vi "MicroDrive Gamepad.vi"() -> ()   [LabVIEW 2012]
uses:
  <vilib>/Utility/miscctls.llb/LVPointTypeDef.ctl
  <vilib>/Utility/inputDevices.llb/closeJoystick.vi
  <vilib>/Utility/inputDevices.llb/joystickAcquire.vi
  MicroDrive.dll
panel:
  in  "m3f":u16(ring)=6 items=["1 X"=1, "2 A"=2, "3 B"=3, "4 Y"=4, "5 LB"=5, "6 RB"=6, "7 LT"=7, "8 RT"=8, "9 Back"=9]
  in  "m3r":u16(ring)=8 items=["1 X"=1, "2 A"=2, "3 B"=3, "4 Y"=4, "5 LB"=5, "6 RB"=6, "7 LT"=7, "8 RT"=8, "9 Back"=9]
  in  "m1f":u16(ring)=3 items=["1 X"=1, "2 A"=2, "3 B"=3, "4 Y"=4, "5 LB"=5, "6 RB"=6, "7 LT"=7, "8 RT"=8, "9 Back"=9]
  out "button selection refs 2":T1
  out "maxVelocityThreeAxis":dbl
  in  "Invert Z":bool=TRUE
  out "Z rev limt":bool
  out "Z Limit":bool
  in  "m3 f":bool
  in  "m3 b":bool
  in  "M3 Velocity":dbl=1.0 format="%.3f"
  in  "M3 Step":dbl=5.0 step=0.1 format="%_6g"
  in  "Reset M3":bool
  out "M3 Axis":dbl format="%.5f"
  in  "closed?":bool
  in  "Slide":cluster{u32, u32, u32}(slide)={7, 6, 2} scale=0.0..7.0
  in  "configure":bool
  in  "device info":bool
  in  "m2f":u16(ring)=4 items=["1 X"=1, "2 A"=2, "3 B"=3, "4 Y"=4, "5 LB"=5, "6 RB"=6, "7 LT"=7, "8 RT"=8, "9 Back"=9]
  in  "halt 3":u16(ring)=9 items=["1 X"=1, "2 A"=2, "3 B"=3, "4 Y"=4, "5 LB"=5, "6 RB"=6, "7 LT"=7, "8 RT"=8, "9 Back"=9]
  in  "m2r":u16(ring)=2 items=["1 X"=1, "2 A"=2, "3 B"=3, "4 Y"=4, "5 LB"=5, "6 RB"=6, "7 LT"=7, "8 RT"=8, "9 Back"=9]
  in  "m1r":u16(ring)=1 items=["1 X"=1, "2 A"=2, "3 B"=3, "4 Y"=4, "5 LB"=5, "6 RB"=6, "7 LT"=7, "8 RT"=8, "9 Back"=9]
  out "X Limit 2":bool
  out "x rev lim":bool
  out "Y Limit 2":bool
  in  "halt 2":bool
  in  "m1 f 2":bool
  in  "m1 b 2":bool
  in  "m2 f 2":bool
  in  "m2 b 2":bool
  out "Y rev lim":bool
  out "Max Velocity One Axis":dbl
  out "Min Velocity":dbl
  in  "Reset All":bool
  in  "Reset M2":bool
  in  "Reset M1":bool
  in  "M2 Step":dbl=5.0 step=0.1 format="%_6g"
  in  "M1 Step":dbl=5.0 step=0.1 format="%_6g"
  in  "M2 Velocity":dbl=1.0 format="%.3f"
  in  "M1 Velocity":dbl=1.0 format="%.3f"
  out "Max VelocityTwo Axis":dbl format="%.3f"
  in  "Invert":bool=TRUE
  in  "Invert":bool
  out "M2 Axis":dbl format="%.5f"
  out "M1 Axis":dbl format="%.5f"
  # "Single Step Controls"
  # "Current Postion"
  # "Step Distances"
  # "mm"
  # "mm"
  # "mm"
  # "mm"
  # "mm"
  # "mm"
  # "Step Velocities"
  # "mm/s"
  # "mm/s"
  # "mm/s"
  # "M3\nControl"
  # "M1\\M2\nControl"
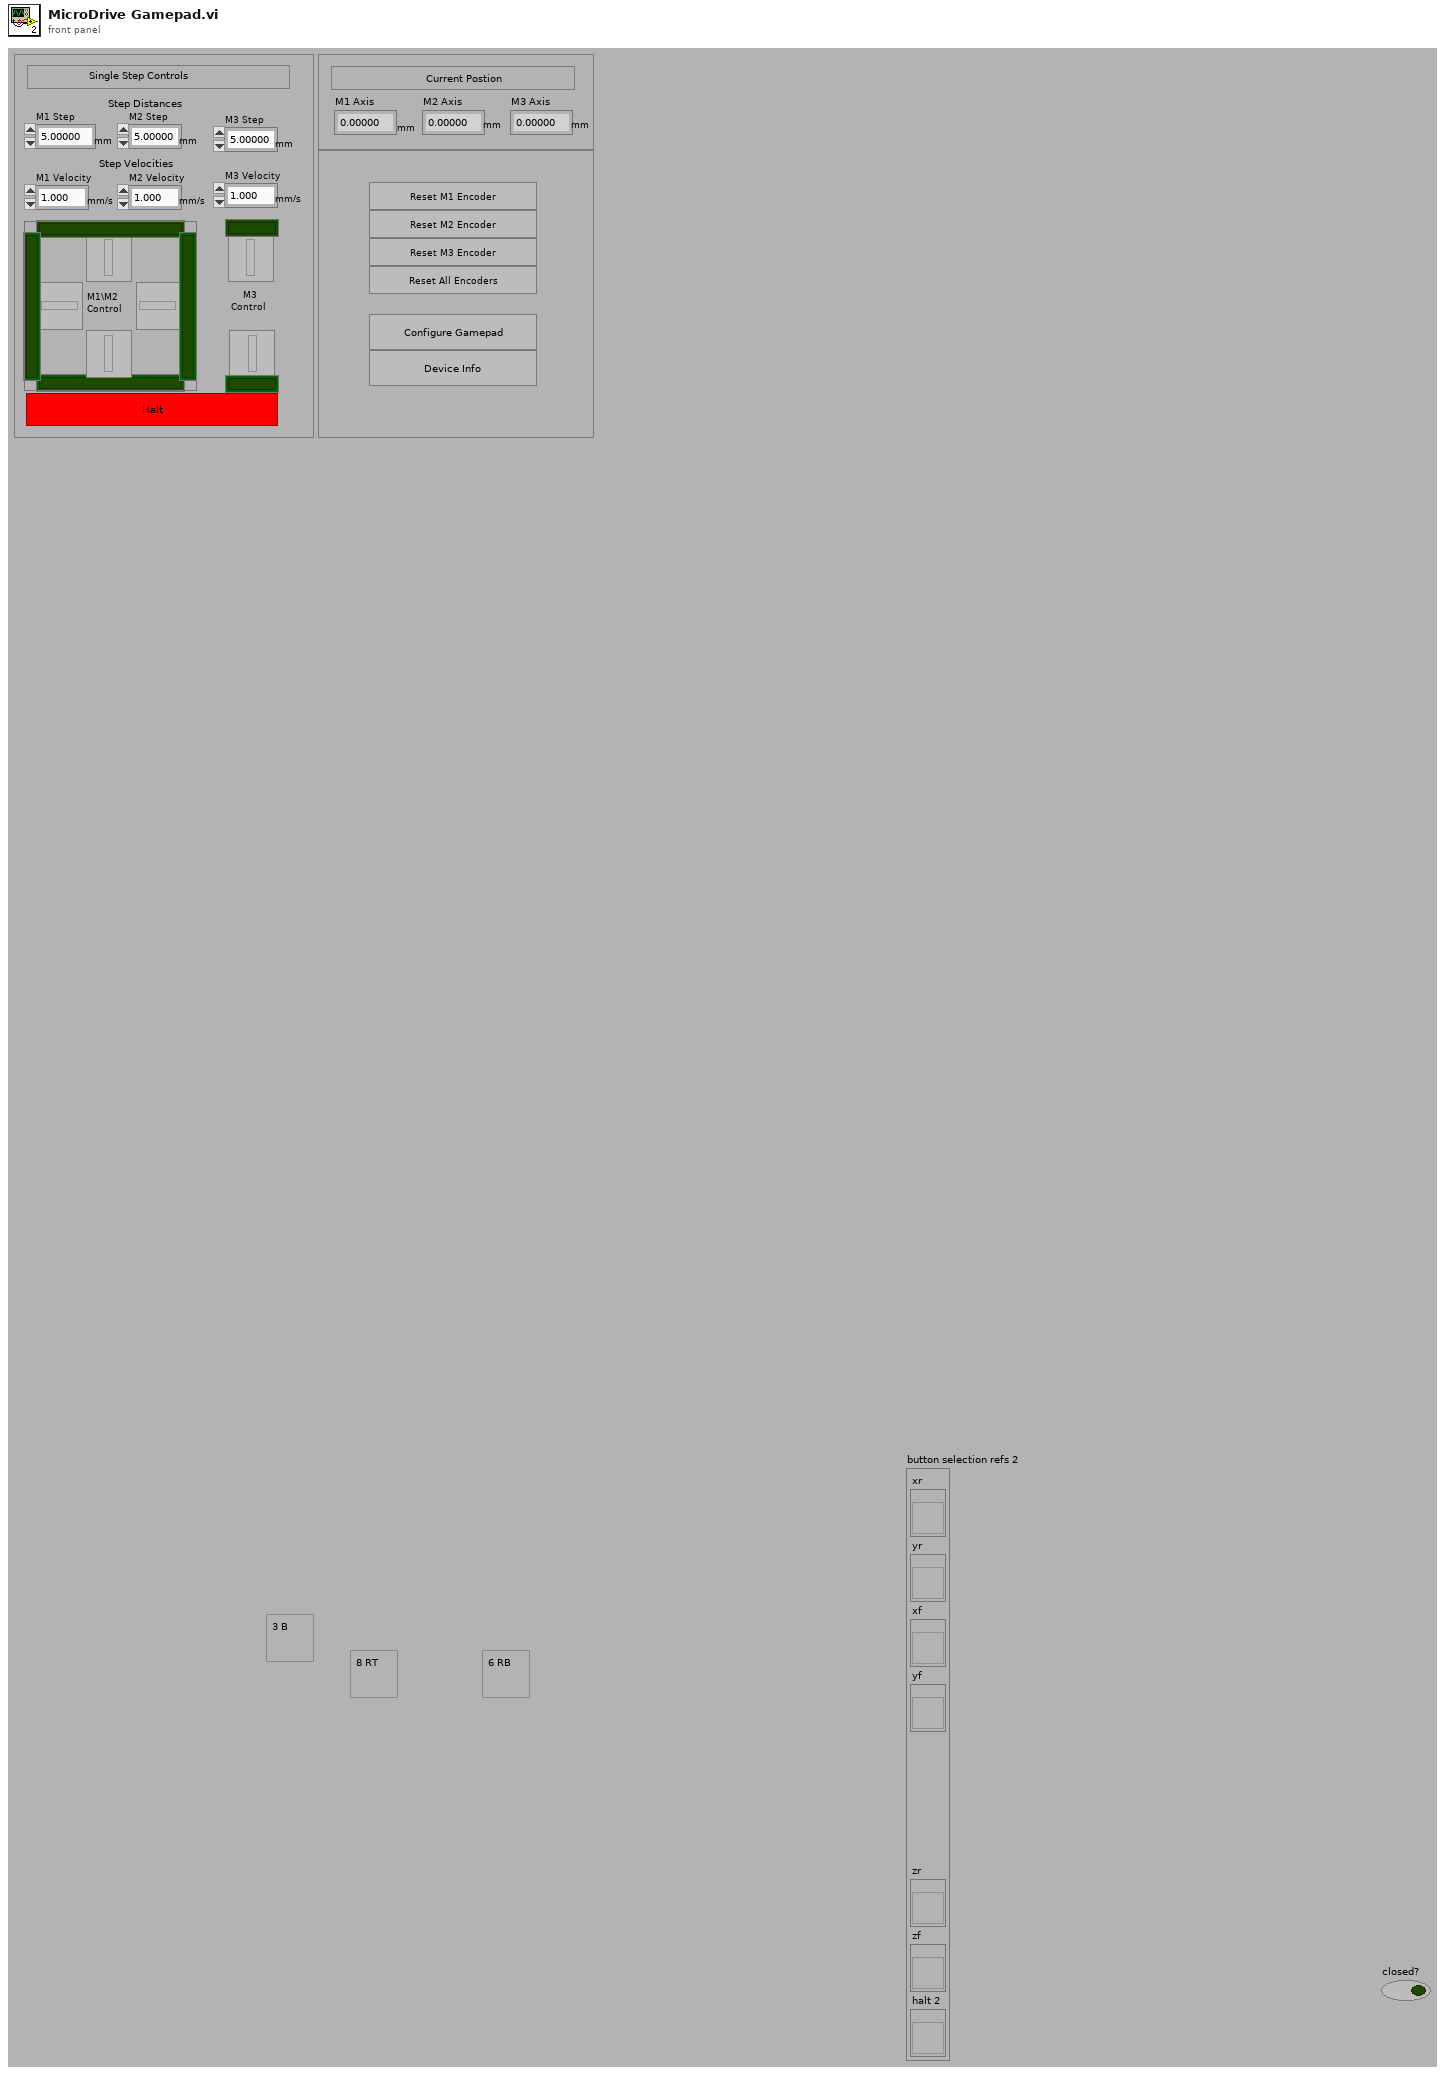
[diagram p1: front panel]
types:
  T1 = cluster{"xr":refnum<vi>, "yr":refnum<vi>, "xf":refnum<vi>, "yf":refnum<vi>, "zr":refnum<vi>, "zf":refnum<vi>, "halt 2":refnum<vi>}
  T2 = typedef "LVPointTypeDef.ctl" = cluster{"Horizontal":i16, "Vertical":i16}
  T3 = cluster{"m1r":refnum<vi>, "m2r":refnum<vi>, "m1f ":refnum<vi>, "m2f":refnum<vi>, "m3r":refnum<vi>, "m3f":refnum<vi>, "halt 3":refnum<vi>}
  T4 = cluster{"X axis":i32, "Y axis":i32, "Z axis":i32, "X axis rotation":i32, "Y axis rotation":i32, "Z axis rotation":i32, "U axis":i32, "V axis":i32}
  T5 = cluster{"button 1":bool, "button 2":bool, "button 3":bool, "button 4":bool, "button 5":bool, "button 6":bool, "button 7":bool, "button 8":bool, "button 9":bool, "button 10":bool, "button 11":bool, "button 12":bool, "button 13":bool, "button 14":bool, "button 15":bool, "button 16":bool, "button 17":bool, "button 18":bool, "button 19":bool, "button 20":bool, "button 21":bool, "button 22":bool, "button 23":bool, "button 24":bool, "button 25":bool, "button 26":bool, "button 27":bool, "button 28":bool, "button 29":bool, "button 30":bool, "button 31":bool, "button 32":bool}
  T6 = cluster{"m1 f 2":bool, "m1 b 2":bool, "m2 f 2":bool, "m2 b 2":bool, "m3 f":bool, "m3 b":bool}
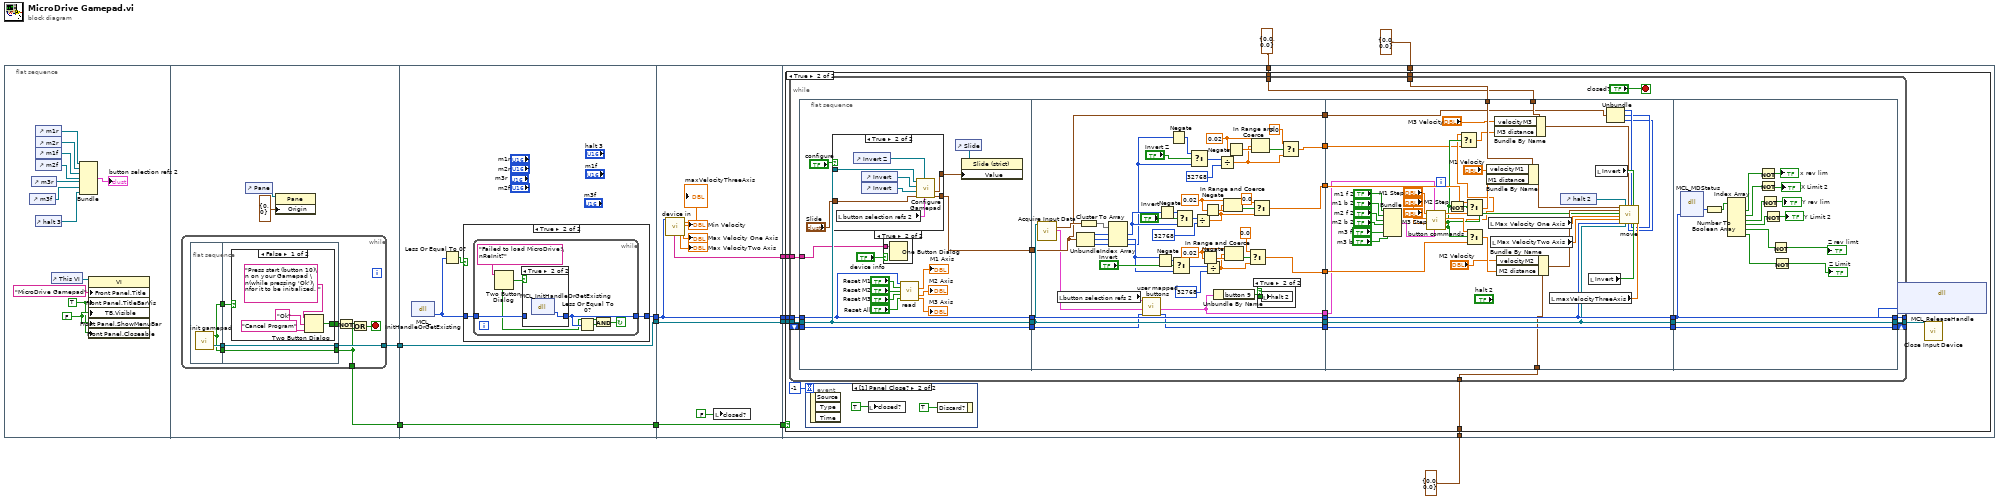
[diagram p0: block diagram]
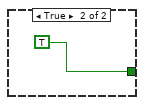
[diagram p2: hidden frame]
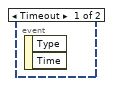
[diagram p6: hidden frame]
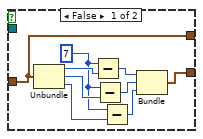
[diagram p8: hidden frame]
diagram:
  n1 = flat-sequence {
    tunnel: [w28] -> w6
    tunnel: [w27] -> w5
    tunnel: [w51] -> w12
    tunnel: [w52] -> w10
    tunnel: [w48] -> w8
    tunnel: w6 -> [w52]
    tunnel: w5 -> [w51]
    tunnel: w12 -> [w71]
    tunnel: [w71] -> w11
    tunnel: w10 -> [w72]
    tunnel: [w72] -> w9
    tunnel: w8 -> [w70]
    tunnel: [w70] -> w7
    tunnel: [w65] -> w4
    tunnel: w7 -> [w77]
    tunnel: w9 -> [w79]
    tunnel: w11 -> [w78]
    tunnel: w4 -> [w76]
    tunnel: cluster{"M1 distance":dbl, "velocityM1":dbl} {"M1 distance"=0.0, "velocityM1"=0.0} ("X Info in") -> [w75]
    tunnel: cluster{"M2 distance":dbl, "velocityM2":dbl} {"M2 distance"=0.0, "velocityM2"=0.0} ("Y Info in") -> [w74]
    tunnel: cluster{"M3 distance":dbl, "velocityM3":dbl} {"M3 distance"=0.0, "velocityM3"=0.0} ("Z Info in") -> [w73]
    frame #0 {
      w18 = TRUE ("Front Panel Window:Closeable")
      w19 = FALSE ("Front Panel Window:Title Bar Visible")
      n2 = control-ref of="m3f"() -> (w13:refnum<vi>)
      n3 = control-ref of="m3r"() -> (w14:refnum<vi>)
      n4 = control-ref of="m1r"() -> (w22:refnum<vi>)
      n5 = control-ref of="m2r"() -> (w23:refnum<vi>)
      n6 = control-ref of="m1f"() -> (w16:refnum<vi>)
      n7 = control-ref of="m2f"() -> (w24:refnum<vi>)
      n8 = control-ref of="halt 3"() -> (w17:refnum<vi>)
      n9 = control-ref of="This VI"() -> (w21:refnum<vi>)
      n10 = Bundle("m1r"=w22, "m2r"=w23, "m1f"=w16, "m2f"=w24, "m3r"=w14, "m3f"=w13, "halt 3"=w17) -> (→"button selection refs 2":T3)  [unwired: 1 out]
      n11 = property class="VI"(reference=w21, "Front Panel.Title"="MicroDrive Gamepad" ("Front Panel Window:Title"), "Front Panel.TitleBarVis"=w18, "TB.Visible"=w19, "Front Panel.ShowMenuBar"=w19, "Front Panel.Closeable"=w18) -> ()  [unwired: 1 in, 2 out]
    }
    frame #1 {
      n12 = while {
        tunnel: [w34] -> w27
        tunnel: [w29] -> w28
        stop <- w33 stop-if-true
        n13 = flat-sequence {
          tunnel: [w37] -> w36
          tunnel: [w38] -> w35
          tunnel: [w37] -> w32
          tunnel: w36 -> [w42]
          tunnel: [w41] -> w34
          tunnel: w35 -> [w41]
          tunnel: [w40] -> w29
          tunnel: w32 -> [w40]
          tunnel: [w39] -> w31
          frame #0 {
            n14 = call "init gamepad.vi"() -> ("device ID"=w38:refnum<k1>, "Joystick found"=w37:bool)  [unwired: 2 out]
          }
          frame #1 {
            n15 = case shown="False" w42 {
              tunnel: [w43 TRUE ("T button?")] -> w39
              frame False {
                n16 = Two Button Dialog(message="Press start (button 10)\n on your Gamepad \n(while pressing 'Ok')\nfor it to be initialized. ", 1:"Cancel Program" ("F button name (\"Cancel\")"), 2:"Ok" ("T button name (\"OK\")")) -> (T button?=w43:bool)
              }
              frame True {
              }
            }
          }
        }
        n17 = Not(x=w31) -> (.not. x?=w30:bool)
        n18 = Or(x=w30, y=w29) -> (x .or. y?=w33:bool)
      }
      n19 = control-ref of="Pane"() -> (w25:refnum<vi>)
      n20 = property class="Pane"(reference=w25, "Origin"=T2 {"Horizontal"=0, "Vertical"=0}) -> ()  [unwired: 1 in, 2 out]
    }
    frame #2 {
      n21 = dll-call lib="C:/Users/Labview/Desktop/SRR/MicroDrive_x64/Labview Examples/MicroDrive.dll" fn="MCL_InitHandleOrGetExisting"() -> ("return type"=w49:i32)  [unwired: 3 in, 2 out]
      n22 = Less Or Equal To 0?(x=w49) -> (x <= 0?=w50:bool)
      n23 = case shown="True" w50 {
        tunnel: w49 -> [w53 w55]
        tunnel: [w53 w54] -> w48
        frame False {
        }
        frame True {
          n24 = while {
            tunnel: w55 -> [w60]
            tunnel: [w58] -> w54
            stop <- w57 continue-if-true
            n25 = Two Button Dialog(message="Failed to load MicroDrive!\nReInit?") -> (T button?=w56:bool)  [unwired: 2 out]
            n26 = case shown="True" w56 {
              tunnel: w60 -> [w62 _]
              tunnel: [w62 w63] -> w58
              frame False {
              }
              frame True {
                n27 = dll-call lib="C:/Users/Labview/Desktop/SRR/MicroDrive_x64/Labview Examples/MicroDrive.dll" fn="MCL_InitHandleOrGetExisting"() -> ("return type"=w63:i32)  [unwired: 3 in, 2 out]
              }
            }
            n28 = Less Or Equal To 0?(x=w58) -> (x <= 0?=w59:bool)
            n29 = And(x=w56, y=w59) -> (x .and. y?=w57:bool)
          }
        }
      }
    }
    frame #3 {
      n30 = call "device in.vi"("handle"=w70) -> ("maxVelocityThreeAxis"=→"maxVelocityThreeAxis":dbl, "Out"=w65:string, "minVelocity"=→"Min Velocity":dbl, "maxVelocityTwoAxis"=→"Max VelocityTwo Axis":dbl, "maxVelocity"=→"Max Velocity One Axis":dbl)  [unwired: 14 out]
      n31 = local write "closed?"(FALSE ("closed?")) -> ()
    }
    frame #4 {
      n32 = case shown="True" w79 {
        tunnel: w78 -> [_ w88]
        tunnel: w77 -> [_ w85]
        tunnel: w76 -> [_ w83]
        tunnel: w75 -> [_ w82]
        tunnel: w74 -> [_ w81]
        tunnel: w73 -> [_ w80]
        frame False {
        }
        frame True {
          n33 = while {
            tunnel: w88 -> [w116]
            tunnel: [w115] -> w87
            tunnel: [w113] -> w86
            tunnel: w85 -> [w111]
            shift-right: [w100] -> _
            shift-left: _ -> [w99]
            tunnel: w83 -> [w97]
            tunnel: w82 -> [w96]
            tunnel: w81 -> [w95]
            tunnel: w80 -> [w94]
            stop <- "closed?" stop-if-true
            n34 = flat-sequence {
              tunnel: [w133] -> w114
              tunnel: [w128] -> w112
              tunnel: [w132] -> w103
              tunnel: w97 -> [w129]
              tunnel: w99 -> [w132]
              tunnel: w111 -> [w128]
              tunnel: w116 -> [w133]
              tunnel: [w118] -> w92
              tunnel: [w195] -> w108
              tunnel: [w198] -> w107
              tunnel: [w197] -> w106
              tunnel: [w196] -> w105
              tunnel: w114 -> [w195]
              tunnel: w112 -> [w198]
              tunnel: [w153] -> w104
              tunnel: w103 -> [w152]
              tunnel: [w176] -> w102
              tunnel: [w173] -> w93
              tunnel: w92 -> [w157]
              tunnel: [w157] -> w91
              tunnel: [w238] -> w110
              tunnel: [w242] -> w109
              tunnel: [w231] -> w101
              tunnel: w102 -> [w231]
              tunnel: w104 -> [w215]
              tunnel: w105 -> [w228]
              tunnel: w106 -> [w227]
              tunnel: w107 -> [w242]
              tunnel: w108 -> [w238]
              tunnel: w96 -> [w225]
              tunnel: w95 -> [w221]
              tunnel: w94 -> [w218]
              tunnel: w93 -> [w209]
              tunnel: w91 -> [w203]
              tunnel: [w246] -> w113
              tunnel: [w260] -> w115
              tunnel: w110 -> [w260]
              tunnel: w109 -> [w246]
              tunnel: w101 -> [w253]
              tunnel: [w253] -> w100
              frame #0 {
                n35 = case shown="True" "configure" {
                  tunnel: w133 -> [_ w149]
                  tunnel: "Slide" -> [w140 w148]
                  tunnel: [w138 w147] -> w118
                  tunnel: [w140 w146] -> w117
                  frame False {
                    w141 = u32 7 ("x")
                    n36 = Unbundle(w140) -> (w142:u32, w143:u32, w139:u32)
                    n37 = Subtract(x=w141, y=w142) -> (x-y=w137:u32)
                    n38 = Subtract(x=w141, y=w143) -> (x-y=w136:u32)
                    n39 = Subtract(x=w141, y=w139) -> (x-y=w135:u32)
                    n40 = Bundle(w137, w136, w135) -> (w138:cluster{u32, u32, u32})  [unwired: 1 in]
                  }
                  frame True {
                    n41 = local read "button selection refs 2"() -> (w144:T1)
                    n42 = control-ref of="Invert Z"() -> (w145:refnum<vi>)
                    n43 = control-ref of="Invert"() -> (w151:refnum<vi>)
                    n44 = control-ref of="Invert"() -> (w150:refnum<vi>)
                    n45 = call "Configure Gamepad.vi"("Cluster 2"=w144, "invert z"=w145, "Slide 3"=w148, "invert y"=w150, "invert x"=w151, "device ID"=w149) -> ("Slide-Function"=w147:cluster{u32, u32, u32}, "Slide Raw"=w146:cluster{u32, u32, u32})  [unwired: 4 out]
                  }
                }
                n46 = case shown="True" "device info" {
                  tunnel: w129 -> [_ w134]
                  frame False {
                  }
                  frame True {
                    n47 = One Button Dialog(message=w134) -> ()  [unwired: 2 out]
                  }
                }
                n48 = call "read.vi"("handle"=w128, "Reset M1"="Reset M1", "Reset M2"="Reset M2", "Reset M3"="Reset M3", "Reset Encoders"="Reset All") -> ("M1 pos"=→"M1 Axis":dbl, "M2 pos"=→"M2 Axis":dbl, "M3 pos"=→"M3 Axis":dbl)  [unwired: 8 in]
                n49 = control-ref of="Slide"() -> (w119:refnum<vi>)
                n50 = property class="Slide (strict)"(reference=w119, "Value"=w117) -> ()  [unwired: 1 in, 2 out]
              }
              frame #1 {
                w169 = 0.02 ("return type")
                w192 = 0.02 ("return type")
                w193 = 0.02 ("return type")
                n51 = call-poly <vilib>:"Acquire Input Data.vi"("device ID"=w195) -> ("axis info"=w178:T4, "button info"=w156:T5)  [unwired: 1 in, 16 out]
                n52 = local read "button selection refs 2"() -> (w154:T1)
                n53 = Unbundle(w157) -> (w160:u32, w159:u32, w158:u32)
                n54 = Cluster To Array(cluster=w178) -> (array=w177:i32[])
                n55 = Index Array(array=w177, index #1=w160, index #2=w159, index #3=w158) -> (element #1=w179:i32, element #2=w174:i32, element #3=w161:i32)
                n56 = call "user mapped buttons.vi"("previous button state"=w152, "gp button info"=w156, "map references"=w154) -> ("current button state"=w176:u32, "gp button info 2"=w153:T5)  [unwired: 7 out]
                n57 = Negate(x=w174) -> (-x=w180:i32)
                n58 = Negate(x=w179) -> (-x=w189:i32)
                n59 = Negate(x=w161) -> (-x=w163:i32)
                n60 = Select(t=w180, s="Invert", f=w174) -> (s? t:f=w190:i32)
                n61 = Select(t=w189, s="Invert", f=w179) -> (s? t:f=w166:i32)
                n62 = Select(t=w163, s="Invert Z", f=w161) -> (s? t:f=w164:i32)
                n63 = Divide(x=w166, y=32768) -> (x/y=w182:dbl)
                n64 = Negate(x=w193) -> (-x=w194:dbl)
                n65 = Negate(x=w192) -> (-x=w191:dbl)
                n66 = Divide(x=w190, y=32768) -> (x/y=w181:dbl)
                n67 = Unbundle By Name(w153) -> ("button 9"=w175:bool)
                n68 = Divide(x=w164, y=32768) -> (x/y=w168:dbl)
                n69 = In Range and Coerce(upper limit=w192, x=w182, lower limit=w191) -> (In Range?=w184:bool)  [unwired: 1 out]
                n70 = In Range and Coerce(upper limit=w193, x=w181, lower limit=w194) -> (In Range?=w186:bool)  [unwired: 1 out]
                n71 = Negate(x=w169) -> (-x=w170:dbl)
                n72 = Select(t=0.0, s=w186, f=w181) -> (s? t:f=w197:dbl)
                n73 = In Range and Coerce(upper limit=w169, x=w168, lower limit=w170) -> (In Range?=w171:bool)  [unwired: 1 out]
                n74 = Select(t=0.0, s=w184, f=w182) -> (s? t:f=w196:dbl)
                n75 = case shown="True" w175 {
                  tunnel: w175 -> [_ w199]
                  frame False {
                  }
                  frame True {
                    n76 = local write "halt 2"(w199) -> ()
                  }
                }
                n77 = Select(t=0.0, s=w171, f=w168) -> (s? t:f=w173:dbl)
              }
              frame #2 {
                n78 = Bundle("m1 f 2"="m1 f 2", "m1 b 2"="m1 b 2", "m2 f 2"="m2 f 2", "m2 b 2"="m2 b 2", "m3 f"="m3 f", "m3 b"="m3 b") -> (w214:T6)  [unwired: 1 out]
                n79 = call "button commands.vi"("Buttons"=w214, "button info"=w215, "M3 Steps"="M3 Step", "M2 Steps"="M2 Step", "M1 Steps"="M1 Step") -> ("Choose Button"=w211:bool, "M3 distance"=w210:dbl, "M2 distance"=w216:dbl, "M1 distance"=w229:dbl)  [unwired: 1 in, 2 out]
                n80 = Not(x=w211) -> (.not. x?=w230:bool)
                n81 = Select(t=w210, s=w211, f=w209) -> (s? t:f=w208:dbl)
                n82 = Select(t=w228, s=w230, f=w229) -> (s? t:f=w224:dbl)
                n83 = Select(t=w216, s=w211, f=w227) -> (s? t:f=w220:dbl)
                n84 = Bundle By Name(cluster=w225, "velocityM1"="M1 Velocity", "M1 distance"=w224) -> (w226:cluster{"M1 distance":dbl, "velocityM1":dbl})
                n85 = local read "Max Velocity One Axis"() -> (w241:dbl)
                n86 = local read "Max VelocityTwo Axis"() -> (w240:dbl)
                n87 = Bundle By Name(cluster=w218, "velocityM3"="M3 Velocity", "M3 distance"=w208) -> (w204:cluster{"M3 distance":dbl, "velocityM3":dbl})
                n88 = Bundle By Name(cluster=w221, "velocityM2"="M2 Velocity", "M2 distance"=w220) -> (w222:cluster{"M2 distance":dbl, "velocityM2":dbl})
                n89 = local read "maxVelocityThreeAxis"() -> (w205:dbl)
                n90 = control-ref of="halt 2"() -> (w232:refnum<vi>)
                n91 = local read "Invert"() -> (w243:bool)
                n92 = local read "Invert"() -> (w239:bool)
                n93 = Unbundle(w203) -> (w202:u32, w201:u32, w200:u32)
                n94 = call "move.vi"("M1 Info in"=w226, "M2 Info in"=w222, "button com"=w211, "max 1"=w241, "max 2"=w240, "handle"=w242, "halt"=w232, "device ID"=w238, "M3 Info in"=w204, "M3 Axis"=w200, "M1 Axis"=w202, "M2 Axis"=w201, "Invert"=w239, "Invert 2"=w243, "max 3"=w205) -> ()  [unwired: 1 in, 4 out]
              }
              frame #3 {
                n95 = dll-call lib="C:/Users/Labview/Desktop/SRR/MicroDrive_x64/Labview Examples/MicroDrive.dll" fn="MCL_MDStatus"("handle"=w246) -> ("status"=w254:u16)  [unwired: 4 in, 4 out]
                n96 = Number To Boolean Array(number=w254) -> (Boolean array=w255:bool[])
                n97 = Index Array(array=w255) -> (element #1=w256:bool, element #2=w257:bool, element #3=w258:bool, element #4=w259:bool, element #5=w248:bool, element #6=w247:bool)  [unwired: 6 in]
                n98 = Not(x=w256) -> (.not. x?=→"x rev lim":bool)
                n99 = Not(x=w257) -> (.not. x?=→"X Limit 2":bool)
                n100 = Not(x=w258) -> (.not. x?=→"Y rev lim":bool)
                n101 = Not(x=w259) -> (.not. x?=→"Y Limit 2":bool)
                n102 = Not(x=w248) -> (.not. x?=→"Z rev limt":bool)
                n103 = Not(x=w247) -> (.not. x?=→"Z Limit":bool)
              }
            }
          }
          n104 = event shown="[1] Panel Close?" {
            selector: _ -> [_ _]
            dyn-events: _ -> [_ _]
            timeout: -1 -> [_ _]
            event Timeout {
              n105 = event-data() -> ()  [unwired: 3 out]
            }
            event Panel Close? {
              n106 = event-data() -> ()  [unwired: 4 out]
              n107 = local write "closed?"(TRUE ("closed?")) -> ()
              n108 = event-data("Discard?"=TRUE) -> ()  [unwired: 1 in, 1 out]
            }
          }
          n109 = dll-call lib="C:/Users/Labview/Desktop/SRR/MicroDrive_x64/Labview Examples/MicroDrive.dll" fn="MCL_ReleaseHandle"("handle"=w86) -> ()  [unwired: 4 in, 3 out]
          n110 = call-poly <vilib>:"Close Input Device.vi"("device ID"=w87) -> ()  [unwired: 1 in, 9 out]
        }
      }
    }
  }
